vi "Initialize.vi"(7 "Serial Configuration":T1={"Baud Rate"=9600, "Parity"=2, "Data Bits"=7} {"Data Bits" items=["7"=7, "8"=8]; "Parity" items=["None", "Odd", "Even"]; "Baud Rate" items=["300"=300, "600"=600, "1200"=1200, "2400"=2400, "4800"=4800, "9600"=9600, "19200"=19200]}, 8 "error in (no error)":errorcluster, 9 "Reset (True)":bool=TRUE, 10 "ID Query (True)":bool=TRUE, 11 "VISA resource name":refnum<visa-resource-name>) -> (0 "error out":errorcluster, 3 "VISA resource name out":refnum<visa-resource-name>)   [LabVIEW 2020, in "Agilent 34401.lvlib"]
doc: "Establishes communication with the instrument and optionally performs an instrument identification query and/or an instrument reset. It also places the instrument in a default state needed for other instrument driver operations. Therefore, call this VI before calling other instrument driver VIs for this instrument. Generally, you need to call the <B>Initialize VI</B> only once at the beginning of an application."
uses:
  <instrlib>/Agilent 34401/Agilent 34401.lvlib
  <instrlib>/Agilent 34401/Private/Extended User Data.ctl
panel:
  # "(c) 2005-2015 National Instruments.  ALL RIGHTS RESERVED."
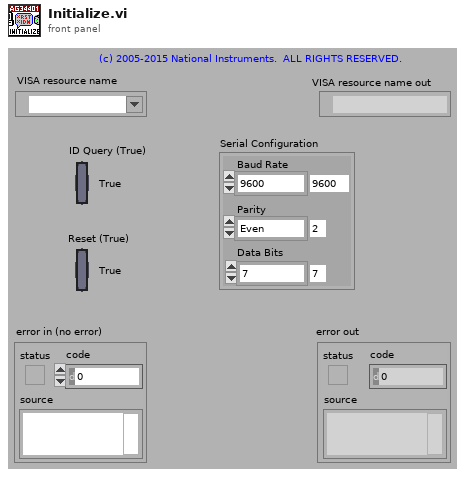
[diagram p1: front panel]
types:
  T1 = cluster{"Baud Rate":u32, "Parity":u16, "Data Bits":u16}
  T2 = typedef "Agilent 34401.lvlib/Extended User Data.ctl" = cluster{"Trigger Source":u16, "Math Storage":u16, "Agilent Model":i32}
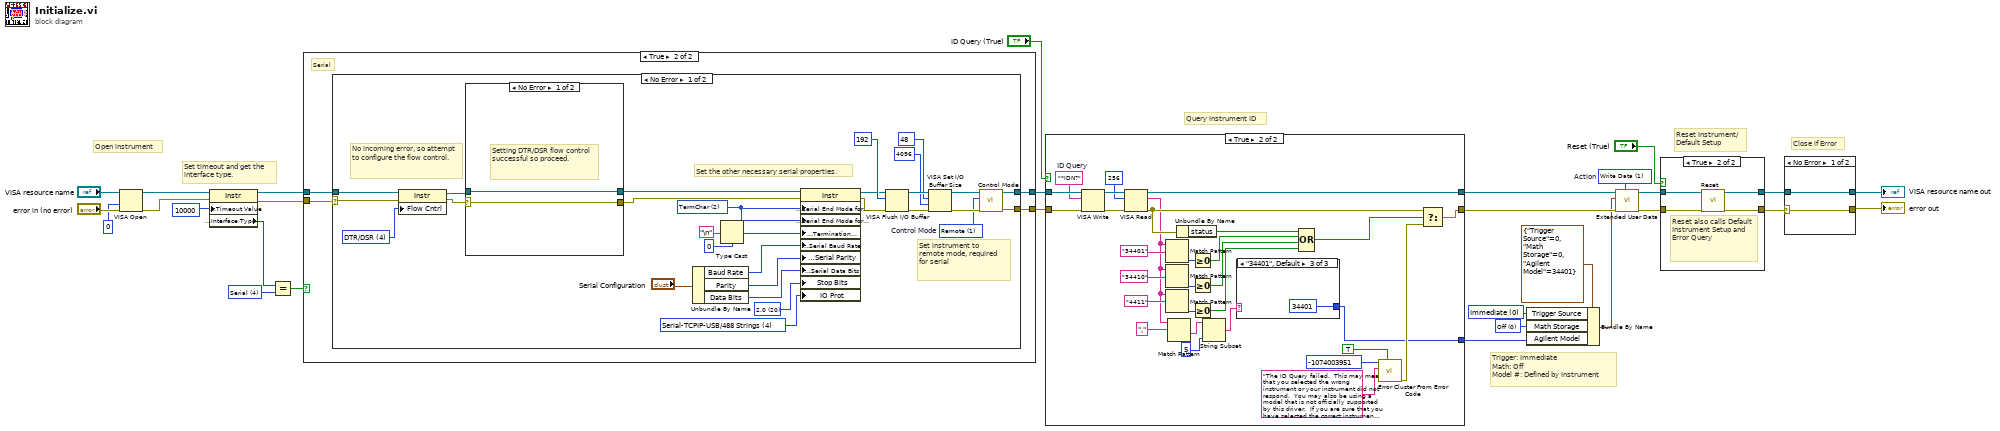
[diagram p0: block diagram]
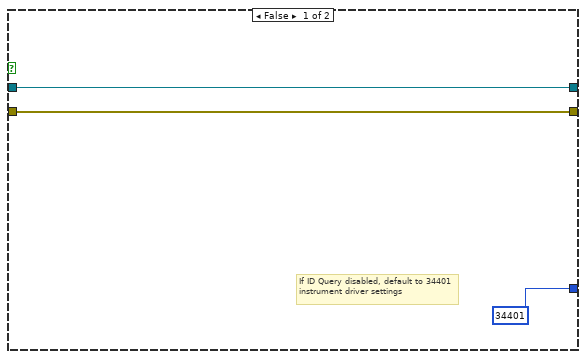
[diagram p2: hidden frame]
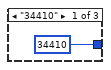
[diagram p3: hidden frame]
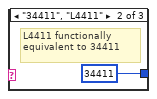
[diagram p4: hidden frame]
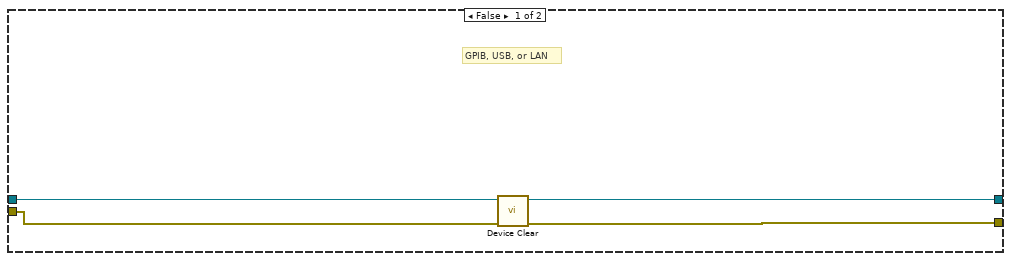
[diagram p5: hidden frame]
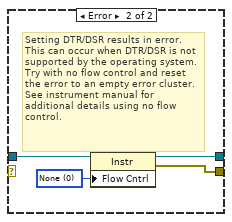
[diagram p6: hidden frame]
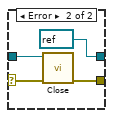
[diagram p8: hidden frame]
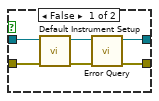
[diagram p9: hidden frame]
diagram:
  w2 = u16 0 items=["Immediate", "Software (Bus)", "External", "Internal"] ("Trigger Source")
  w3 = u16 0 items=["Off", "Internal Buffer", "Output Buffer"] ("Math Storage")
  w6 = u16 1 items=["Read Data", "Write Data", "Dispose of Data"]  # Action
  w23 = u16 4 items=["GPIB"=1, "VXI"=2, "GPIB-VXI"=3, "Serial"=4, "PXI"=5, "TCPIP"=6, "USB"=7] ("Interface Information:Interface Type")
  # "Trigger: Immediate\nMath: Off\nModel #: Defined by Instrument"
  # "Set timeout and get the\ninterface type."
  # "Close if Error"
  # "Query Instrument ID"
  # "Reset Instrument/\nDefault Setup"
  # "Open instrument"
  n1 = VISA Open(access mode=u32 0, error in (no error)="error in (no error)", VISA resource name="VISA resource name") -> (VISA resource name=w14:refnum<visa-resource-name>, error out=w13:errorcluster)  [unwired: 2 in]
  n2 = property on="Property Node" class="Instr"(reference=w14, error in=w13, "General Settings:Timeout Value"=u32 10000) -> (reference out=w12:refnum<visa-resource-name>, error out=w11:errorcluster, "Interface Information:Interface Type"=w26:u16)
  n3 = Equal?(x=w26, y=w23) -> (x = y?=w24:bool)
  n4 = case shown="True" w24 {
    tunnel: [w31 w37] -> w17
    tunnel: [w30 w36] -> w15
    tunnel: w12 -> [w32 w35]
    tunnel: w11 -> [w33 w34]
    frame False {
      # "GPIB, USB, or LAN"
      n5 = call <instrlib>:"Device Clear.vi"("error in (no error)"=w33, "VISA Resource Name"=w32) -> ("error out"=w30:errorcluster, "VISA Resource Out"=w31:refnum<visa-resource-name>)  [unwired: 8 in]
    }
    frame True {
      # "Serial"
      n6 = case shown="No Error" w34 {
        selector: w34 -> [w38 w73]
        tunnel: [w59 w74] -> w37
        tunnel: [w58 w73] -> w36
        tunnel: w35 -> [w55 w74]
        frame No Error {
          w52 = u16 4 items=["Normal"=1, "VXI/FDC"=2, "GPIB/HS488"=3, "Serial-TCPIP-USB/488 Strings"=4, "USBTMC/Vendor-Specific"=5] ("Message Based Settings:IO Protocol")
          w51 = u16 20 items=["1.0"=10, "1.5"=15, "2.0"=20] ("Serial Settings:Serial Stop Bits")
          w45 = u16 2 items=["None", "LastBit", "TermChar"] ("Serial Settings:Serial End Mode for Reads")
          w57 = u16 1 items=["Local", "Remote", "Remote with Lock"]  # Control Mode
          w56 = u16 4 items=["None", "XON/XOFF", "RTS/CTS", "XON/XOFF & RTS/CTS", "DTR/DSR", "XON/XOFF & DTR/DSR"] ("Serial Settings:Serial Flow Control")
          # "Set the other necessary serial properties."
          # "No incoming error, so attempt to configure the flow control."
          # "Set instrument to remote mode, required for serial"
          n7 = property on="Property Node" class="Instr"(reference=w55, error in=w38, "Flow Cntrl"=w56) -> (reference out=w54:refnum<visa-resource-name>, error out=w53:errorcluster)
          n8 = case shown="No Error" w53 {
            selector: w53 -> [w67 _]
            tunnel: w54 -> [w68 w69]
            tunnel: [w68 w70] -> w41
            tunnel: [w67 w71] -> w42
            frame No Error {
              # "Setting DTR/DSR flow control successful so proceed."
            }
            frame Error {
              w72 = u16 0 items=["None", "XON/XOFF", "RTS/CTS", "XON/XOFF & RTS/CTS", "DTR/DSR", "XON/XOFF & DTR/DSR"] ("Serial Settings:Serial Flow Control")
              # "Setting DTR/DSR results in error. This can occur when DTR/DSR is not supported by the operating system.  Try with no flow control and reset the error to an empty error cluster. See instrument manual for additional details using no flow control."
              n9 = property on="Property Node" class="Instr"(reference=w69, "Flow Cntrl"=w72) -> (reference out=w70:refnum<visa-resource-name>, error out=w71:errorcluster)  [unwired: 1 in]
            }
          }
          n10 = Unbundle By Name("Serial Configuration") -> ("Baud Rate"=w48:u32, "Parity"=w50:u16, "Data Bits"=w49:u16)
          n11 = Type Cast(type=u8 0, x="\n" ("Line Feed Constant")) -> (*(type *) &x=w46:u8)
          n12 = property on="Property Node" class="Instr"(reference=w41, error in=w42, "Serial Settings:Serial End Mode for Reads"=w45, "Serial Settings:Serial End Mode for Writes"=w45, "Message Based Settings:Termination Character"=w46, "Serial Settings:Serial Baud Rate"=w48, "Serial Settings:Serial Parity"=w50, "Serial Settings:Serial Data Bits"=w49, "Stop Bits"=w51, "IO Prot"=w52) -> (reference out=w40:refnum<visa-resource-name>, error out=w39:errorcluster)
          n13 = VISA Flush I/O Buffer(VISA resource name=w40, mask (16)=u16 192, error in (no error)=w39) -> (VISA resource name out=w66:refnum<visa-resource-name>, error out=w65:errorcluster)
          n14 = VISA Set I/O Buffer Size(VISA resource name=w66, mask (16)=u16 48, size (4096)=u32 4096 ("size (0)"), error in (no error)=w65) -> (VISA resource name out=w61:refnum<visa-resource-name>, error out=w60:errorcluster)
          n15 = call <instrlib>:"Control Mode.vi"("error in (no error)"=w60, "Control Mode (0:Local)"=w57, "VISA Resource Name"=w61) -> ("error out"=w58:errorcluster, "VISA Resource Out"=w59:refnum<visa-resource-name>)  [unwired: 7 in]
        }
        frame Error {
          # "If there is an error in, do not attempt to set additional serial parameters."
        }
      }
    }
  }
  n16 = case shown="True" "ID Query (True)" {
    tunnel: [w76 w107] -> w9
    tunnel: [w77 w104] -> w8
    tunnel: w17 -> [w77 w105]
    tunnel: w15 -> [w76 w106]
    tunnel: [34401 w78] -> w4
    frame False {
      # "If ID Query disabled, default to 34401 instrument driver settings"
    }
    frame True {
      w99 = "*IDN?"  # ID Query
      n17 = VISA Write(VISA resource name=w105, write buffer=w99, error in (no error)=w106) -> (VISA resource name out=w103:refnum<visa-resource-name>, error out=w102:errorcluster)  [unwired: 1 out]
      n18 = VISA Read(VISA resource name=w103, byte count=u32 256, error in (no error)=w102) -> (VISA resource name out=w104:refnum<visa-resource-name>, read buffer=w80:string, error out=w93:errorcluster)  [unwired: 1 out]
      n19 = Match Pattern(string=w80, regular expression="34401") -> (offset past match=w94:i32)  [unwired: 1 in, 3 out]
      n20 = Match Pattern(string=w80, regular expression="34410") -> (offset past match=w91:i32)  [unwired: 1 in, 3 out]
      n21 = Match Pattern(string=w80, regular expression="4411") -> (offset past match=w90:i32)  [unwired: 1 in, 3 out]
      n22 = Match Pattern(string=w80, regular expression=",") -> (after substring=w82:string)  [unwired: 1 in, 3 out]
      n23 = Unbundle By Name(w93) -> ("status"=w92:bool)
      n24 = Greater Or Equal To 0?(x=w94) -> (x >= 0?=w87:bool)
      n25 = Greater Or Equal To 0?(x=w91) -> (x >= 0?=w86:bool)
      n26 = Greater Or Equal To 0?(x=w90) -> (x >= 0?=w85:bool)
      n27 = String Subset(string=w82, length (rest)=5 ("length (rest)")) -> (substring=w79:string)  [unwired: 1 in]
      n28 = case shown="\"34401\", Default" w79 {
        tunnel: [34410 ("number 3") 34411 ("number 3") 34401 ("number 3")] -> w78
        frame "34410" {
        }
        frame "34411", "L4411" {
          # "L4411 functionally equivalent to 34411"
        }
        frame "34401", Default {
        }
      }
      n29 = Compound Arithmetic op=OR(w92, w87, w86, w85) -> (w84:bool)
      n30 = call <vilib>:"Error Cluster From Error Code.vi"("show call chain? (False)"=TRUE, "error message (\"\")"="The ID Query failed.  This may mean that you selected the wrong instrument or your instrument did not respond.  You may also be using a model that is not officially supported by this driver.  If you are sure that you have selected the correct instrument and it is responding, try disabling the ID Query." ("Source (VI Name)"), "error code (0)"=-1074003951 ("Code")) -> ("error out"=w98:errorcluster)  [unwired: 6 in]
      n31 = Select(t=w93, s=w84, f=w98) -> (s? t:f=w107:errorcluster)
    }
  }
  n32 = Bundle By Name(cluster=T2 {"Trigger Source"=0, "Math Storage"=0, "Agilent Model"=34401} ("User Data Definition"), "Trigger Source"=w2, "Math Storage"=w3, "Agilent Model"=w4) -> (w1:T2)
  n33 = call <instrlib>:"Extended User Data.vi"("Action (0: Read Data)"=w6, "Error In (no error)"=w9, "User Data In"=w1, "VISA resource name in"=w8) -> ("Error Out"=w10:errorcluster, "VISA resource name out"=w7:refnum<visa-resource-name>)  [unwired: 5 in, 1 out]
  n34 = case shown="True" "Reset (True)" {
    tunnel: w10 -> [w115 w117]
    tunnel: [w112 w120] -> w19
    tunnel: w7 -> [w116 w118]
    tunnel: [w111 w119] -> w20
    frame False {
      n35 = call <instrlib>:"Default Instrument Setup.vi"("error in (no error)"=w115, "VISA resource name"=w116) -> ("error out"=w113:errorcluster, "VISA resource name out"=w114:refnum<visa-resource-name>)  [unwired: 8 in]
      n36 = call <instrlib>:"Error Query.vi"("error in (no error)"=w113, "VISA resource name"=w114) -> ("error out"=w112:errorcluster, "VISA resource name out"=w111:refnum<visa-resource-name>)  [unwired: 6 in, 2 out]
    }
    frame True {
      # "Reset also calls Default Instrument Setup and Error Query"
      n37 = call <instrlib>:"Reset.vi"("error in (no error)"=w117, "VISA resource name"=w118) -> ("error out"=w120:errorcluster, "VISA resource name out"=w119:refnum<visa-resource-name>)  [unwired: 8 in]
    }
  }
  n38 = case shown="No Error" w19 {
    selector: w19 -> [w121 w124]
    tunnel: w20 -> [w122 w125]
    tunnel: [w122 refnum<visa-resource-name> refnum ("VISA resource name out")] -> w21
    tunnel: [w121 w126] -> w16
    frame No Error {
    }
    frame Error {
      n39 = call <instrlib>:"Close.vi"("error in (no error)"=w124, "VISA resource name"=w125) -> ("error out"=w126:errorcluster)  [unwired: 9 in]
    }
  }
  "VISA resource name out" <- w21
  "error out" <- w16
